vi "getting_started_SynchronizationSaveTestWithTimer.vi"() -> ()   [LabVIEW 2019]
uses:
  C:/Users/Mastlab/Desktop/IMU VectorNAV VI/VectorNav.dll
  VectorNav.dll
panel:
  in  "Path":path
  out "Timer":dbl
  out "Ready":bool
  out "Ending":bool
  out "Queue #":dbl
  in  "stop":bool
  out "Async Enable":bool
  out "Sensor Connected":bool
  out "Accel.Z":sgl
  out "Accel.Y":sgl
  out "Accel.X":sgl
  out "Gyro.Z":sgl
  out "Gyro.Y":sgl
  out "Gyro.X":sgl
  in  "Baudrate":string="115200"
  in  "COM Port":string="COM1"
  # "Note: Wait for 'Ready' to light up\nNote: Start Motion whitin 10 seconds after starting this VI"
  # "Data"
  # "Diagnostics"
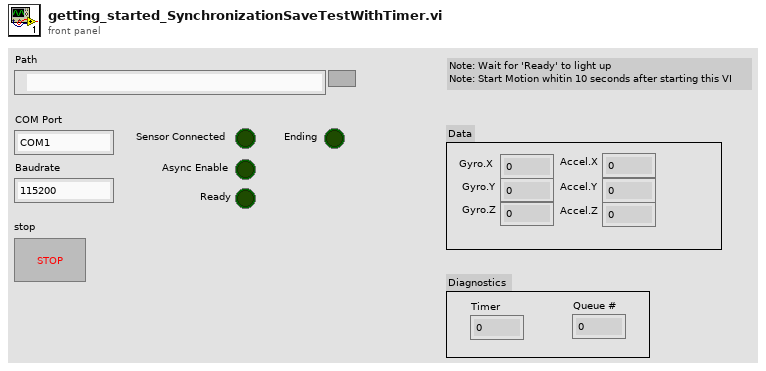
[diagram p1: front panel]
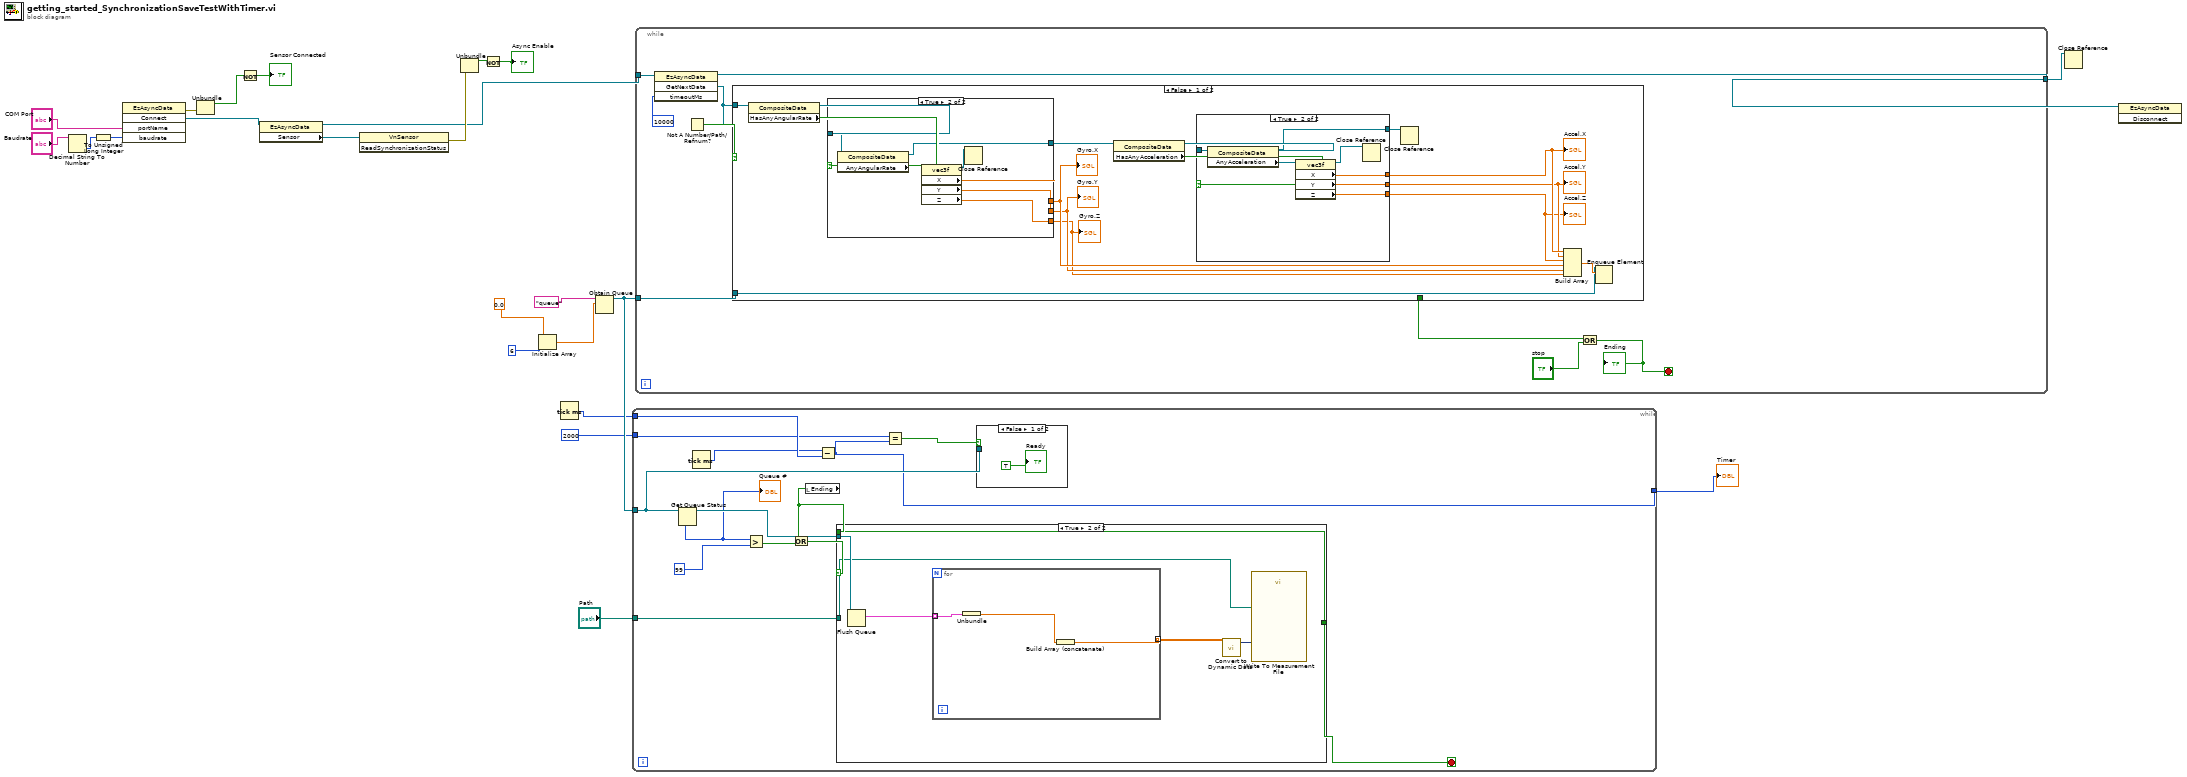
[diagram p0: block diagram]
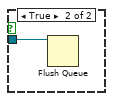
[diagram p2: hidden frame]
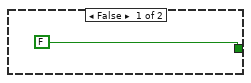
[diagram p3: hidden frame]
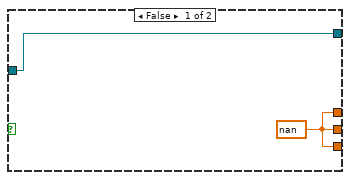
[diagram p4: hidden frame]
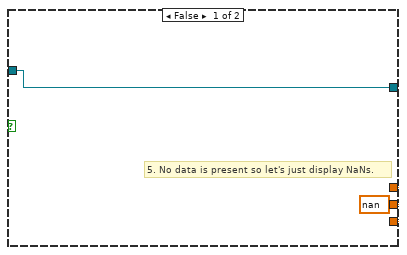
[diagram p5: hidden frame]
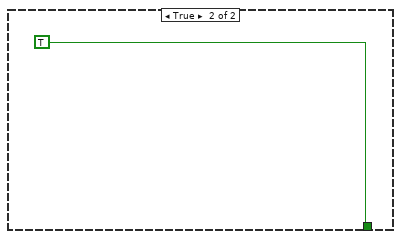
[diagram p6: hidden frame]
diagram:
  n1 = Decimal String To Number(string="Baudrate") -> (number=w23:i32)  [unwired: 2 in, 1 out]
  n2 = To Unsigned Long Integer(number=w23) -> (unsigned 32bit integer=w21:u32)
  n3 = invoke class="EzAsyncData" method="Connect"("portName"="COM Port", "baudrate"=w21) -> (error out=w19:errorcluster, "Connect"=w17:refnum<k24>)  [unwired: 3 in, 3 out]
  n4 = Unbundle(w19) -> ("status"=w18:bool)  [unwired: 2 out]
  n5 = Not(x=w18) -> (.not. x?=→"Sensor Connected":bool)
  n6 = property class="EzAsyncData"(reference=w17) -> (reference out=w5:refnum<k24>, "Sensor"=w16:refnum<k24>)  [unwired: 1 in, 1 out]
  n7 = invoke class="VnSensor" method="ReadSynchronizationStatus"(reference=w16) -> (error out=w15:errorcluster)  [unwired: 2 in, 2 out]
  n8 = Unbundle(w15) -> ("status"=w14:bool)  [unwired: 2 out]
  n9 = Not(x=w14) -> (.not. x?=→"Async Enable":bool)
  n10 = Initialize Array(0.0, 6) -> (w10:dbl[])
  n11 = Tick Count (ms)() -> (millisecond timer value=w3:u32)
  n12 = Obtain Queue(name (unnamed)="queue", element data type=w10) -> (queue out=w7:refnum<queue>)  [unwired: 3 in, 2 out]
  n13 = while {
    tunnel: w7 -> [w27]
    tunnel: 2000 -> [w28]
    tunnel: w3 -> [w30]
    tunnel: [w25] -> w2
    tunnel: "Path" -> [w24]
    stop <- w32 stop-if-true
    n14 = Get Queue Status(queue=w27) -> (queue out=w36:refnum<queue>, # elements in queue=w35:i32)  [unwired: 2 in, 6 out]
    "Queue #" <- w35
    n15 = Tick Count (ms)() -> (millisecond timer value=w29:u32)
    n16 = Greater?(x=w35, y=99) -> (0:w33:bool)
    n17 = local read "Ending"() -> (w31:bool)
    n18 = Or(x=w31, y=w33) -> (x .or. y?=w34:bool)
    n19 = Subtract(x=w29, y=w30) -> (x-y=w25:u32)
    n20 = case shown="True" w34 {
      tunnel: w36 -> [_ w46]
      tunnel: [FALSE w42] -> w32
      tunnel: w31 -> [_ w42]
      tunnel: w24 -> [_ w41]
      frame False {
      }
      frame True {
        n21 = Flush Queue(queue=w46) -> (remaining elements=w45:cluster{dbl[]}[])  [unwired: 1 in, 2 out]
        n22 = for {
          tunnel: w45 -> [w48] mode=indexing
          tunnel: [w49] -> w43 mode=indexing
          n23 = Unbundle(w48) -> (w47:dbl[])
          n24 = Build Array (concatenate)(w47) -> (w49:dbl[])
        }
        n25 = call "Convert to Dynamic Data"("2D Array"=w43) -> ("Dynamic Data Type"=w44:dynamicdata)  [unwired: 3 in]
        n26 = call "Write To Measurement File"("Signals"=w44, "Filename"=w41) -> ()  [unwired: 15 in, 3 out]
      }
    }
    n27 = Equal?(x=w28, y=w25) -> (x = y?=w26:bool)
    n28 = case shown="False" w26 {
      tunnel: w27 -> [_ w39]
      frame False {
        "Ready" <- TRUE
      }
      frame True {
        n29 = Flush Queue(queue=w39) -> ()  [unwired: 1 in, 3 out]
      }
    }
  }
  "Timer" <- w2
  n30 = while {
    tunnel: [w58] -> w12
    tunnel: w7 -> [w56]
    tunnel: w5 -> [w53]
    stop <- w54 stop-if-true
    n31 = invoke class="EzAsyncData" method="GetNextData"(reference=w53, "timeoutMs"=10000) -> (reference out=w58:refnum<k24>, "GetNextData"=w50:refnum<k24>)  [unwired: 2 in, 2 out]
    n32 = Not A Number/Path/Refnum?(number/path/refnum=w50) -> (NaN/Path/Refnum?=w51:bool)
    n33 = case shown="False" w51 {
      tunnel: w50 -> [w67 _]
      tunnel: [_ TRUE] -> w55
      tunnel: w56 -> [w63 _]
      frame False {
        n34 = property on="Property Node" class="CompositeData"(reference=w67) -> (reference out=w71:refnum<k24>, "HasAnyAngularRate"=w72:bool)  [unwired: 1 in, 1 out]
        n35 = case shown="True" w72 {
          tunnel: w71 -> [w83 w86]
          tunnel: [w84 w87] -> w61
          tunnel: [w84 w88] -> w60
          tunnel: [w84 w89] -> w59
          tunnel: [w83 w91] -> w70
          frame False {
            w84 = sgl nan
            # "5. No data is present so let's just display NaNs."
          }
          frame True {
            n36 = property class="CompositeData"(reference=w86) -> (reference out=w91:refnum<k24>, "AnyAngularRate"=w85:refnum<k24>)  [unwired: 1 in, 1 out]
            n37 = property class="vec3f"(reference=w85) -> (reference out=w90:refnum<k24>, "X"=w87:sgl, "Y"=w88:sgl, "Z"=w89:sgl)  [unwired: 1 in, 1 out]
            n38 = Close Reference(reference=w90) -> ()  [unwired: 1 in, 1 out]
          }
        }
        "Gyro.X" <- w61
        "Gyro.Y" <- w60
        "Gyro.Z" <- w59
        n39 = property class="CompositeData"(reference=w70) -> (reference out=w68:refnum<k24>, "HasAnyAcceleration"=w69:bool)  [unwired: 1 in, 1 out]
        n40 = case shown="True" w69 {
          tunnel: w68 -> [w74 w82]
          tunnel: [w75 w77] -> w66
          tunnel: [w75 w78] -> w65
          tunnel: [w75 w79] -> w62
          tunnel: [w74 w81] -> w73
          frame False {
            w75 = sgl nan
          }
          frame True {
            n41 = property class="CompositeData"(reference=w82) -> (reference out=w81:refnum<k24>, "AnyAcceleration"=w80:refnum<k24>)  [unwired: 1 in, 1 out]
            n42 = property class="vec3f"(reference=w80) -> (reference out=w76:refnum<k24>, "X"=w77:sgl, "Y"=w78:sgl, "Z"=w79:sgl)  [unwired: 1 in, 1 out]
            n43 = Close Reference(reference=w76) -> ()  [unwired: 1 in, 1 out]
          }
        }
        "Accel.X" <- w66
        "Accel.Y" <- w65
        "Accel.Z" <- w62
        n44 = Close Reference(reference=w73) -> ()  [unwired: 1 in, 1 out]
        n45 = Build Array(w66, w65, w62, w61, w60, w59) -> (w64:sgl[])
        n46 = Enqueue Element(queue=w63, element=w64) -> ()  [unwired: 2 in, 3 out]
      }
      frame True {
      }
    }
    n47 = Or(x=w55, y="stop") -> (x .or. y?=w54:bool)
    "Ending" <- w54
  }
  n48 = Close Reference(reference=w12) -> ()  [unwired: 1 in, 1 out]
  n49 = invoke class="EzAsyncData" method="Disconnect"(reference=w12) -> ()  [unwired: 2 in, 3 out]
